vi "test_vision.vi"() -> ()   [LabVIEW 2011]
uses:
  Vision Instrumentation Control.ctl
  <vilib>/vision/NI_Vision_Development_Module.lvlib
panel:
  out "Exe Times":u32[](array[numeric])
  out "Total Execution Time":u32
  out "Avg Execution Time":dbl
  in  "Range":cluster{"Lower value":sgl, "Upper value":sgl}={"Lower value"=218.04347, "Upper value"=255.0} {"Lower value" scale=0.0..255.0; "Upper value" scale=0.0..255.0}
  in  "Score Limits":T1={"Rect Coverage"=76.0, "Aspect Ratio"=0.0, "X Edge Strength"=40.0, "Y Edge Strength"=50.0}
  in  "Area Size Limit":i32=444
  in  "Particle Count Limit":i32=8
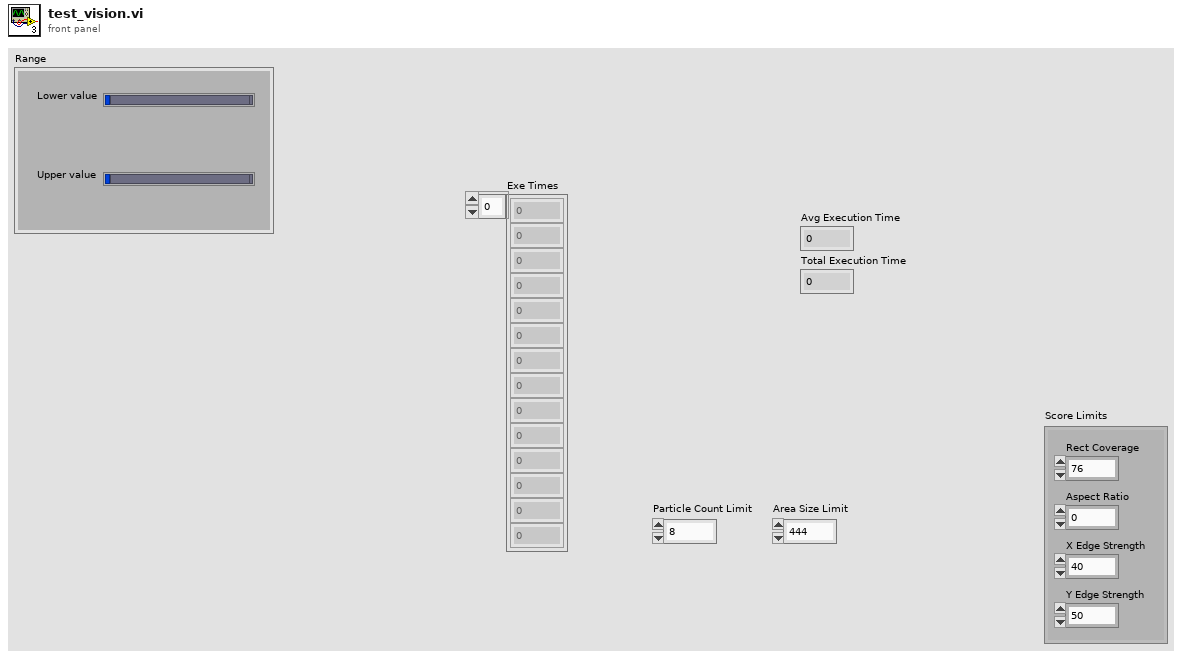
[diagram p1: front panel]
types:
  T1 = cluster{"Rect Coverage":dbl, "Aspect Ratio":dbl, "X Edge Strength":dbl, "Y Edge Strength":dbl}
  T2 = typedef "Image Type" = u32
  T3 = typedef "IMAQ Image.ctl" = refnum<image>
  T4 = typedef "Vision Instrumentation Control.ctl" = cluster{"Draw Boxes":bool, "Draw Scores":bool, "Draw Lines":bool, "Draw Line Angles":bool, "Draw Targets":bool, "Draw Compound Crosshair":bool, "Draw Center Line":bool}
  T5 = enum32{"AutoM", "Close", "Dilate", "Erode", "Gradient", "Gradient in", "Gradient out", "HitMiss", "Open", "PClose", "POpen", "Thick", "Thin"}
  T6 = enum32{"AutoM", "Close", "Dilate", "Erode", "Gradient", "Gradient out", "Gradient in", "Hit miss", "Open", "PClose", "POpen", "Thick", "Thin"}
  T7 = cluster{cluster{"Left":dbl, "Top":dbl, "Right":dbl, "Bottom":dbl}, cluster{"Score":dbl, "Score":dbl, "X Score":dbl, "Y Score":dbl}, "Clipped Edge":cluster{"Left":bool, "Top":bool, "Right":bool, "Bottom":bool}}[]
  T8 = typedef "Camera State.ctl" = enum16{"No Targets", "Low Confidence", "Medium Confidence", "High Confidence", "Camera Error"}
  T9 = cluster{"X Position":dbl, "Distance":dbl, "Camera State":T8}
  T10 = typedef "Diamond Target Output.ctl" = cluster{"Position":cluster{"X":dbl, "Y":dbl, "Distance":dbl}, "Est. Position":T11, "Target Confidence":T12}
  T11 = typedef "Rectangle Position.ctl" = enum16{"Unknown", "Top", "Right", "Left", "Bottom"}
  T12 = typedef "Target Confidence.ctl" = enum16{"Good", "Good-Clipped Y", "Marginal-Clipped X"}
  T13 = typedef "Line.ctl" = cluster{"First Point":cluster{"X":dbl, "Y":dbl, "Index":dbl}, "Second Point":cluster{"X":dbl, "Y":dbl, "Index":dbl}, "theta":dbl, "Direction":T14, "Line Confidence":T15}
  T14 = typedef "Direction.ctl" = enum16{"Rt", "Rt-Up", "Up", "Lt-Up", "Lt", "Lt-Dn", "Dn", "Rt-Dn", "Unknown"}
  T15 = typedef "Line Confidence.ctl" = enum16{"Good", "Bad"}
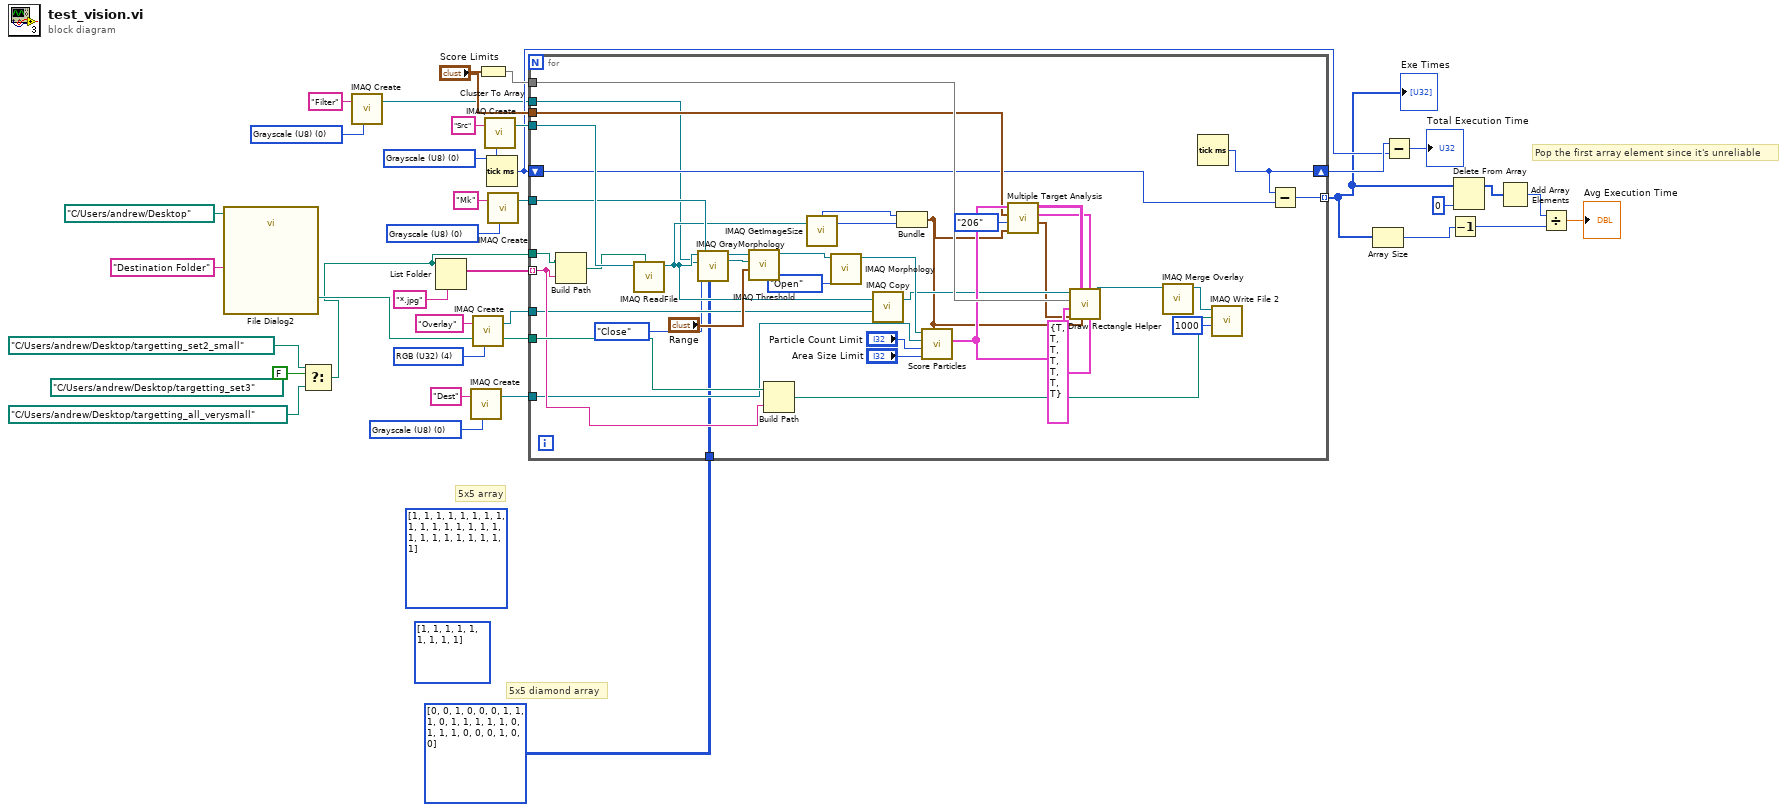
[diagram p0: block diagram]
diagram:
  (unwired) i32[][] [[1, 1, 1], [1, 1, 1], [1, 1, 1]] ("Structuring Element")
  (unwired) i32[][] [[1, 1, 1, 1, 1], [1, 1, 1, 1, 1], [1, 1, 1, 1, 1], [1, 1, 1, 1, 1], [1, 1, 1, 1, 1]] ("Structuring Element")
  w4 = T2 0 items=["Grayscale (U8)", "Grayscale (I16)", "Grayscale (SGL)", "Complex (CSG)", "RGB (U32)", "HSL (U32)", "RGB (U64)", "Grayscale (U16)"] ("Image Type")
  w17 = T2 4 items=["Grayscale (U8)", "Grayscale (I16)", "Grayscale (SGL)", "Complex (CSG)", "RGB (U32)", "HSL (U32)", "RGB (U64)", "Grayscale (U16)"] ("Image Type")
  (unwired) path "C:/Users/andrew/Desktop/targetting_set3" ("path")
  w23 = T2 0 items=["Grayscale (U8)", "Grayscale (I16)", "Grayscale (SGL)", "Complex (CSG)", "RGB (U32)", "HSL (U32)", "RGB (U64)", "Grayscale (U16)"] ("Image Type")
  w31 = T2 0 items=["Grayscale (U8)", "Grayscale (I16)", "Grayscale (SGL)", "Complex (CSG)", "RGB (U32)", "HSL (U32)", "RGB (U64)", "Grayscale (U16)"] ("Image Type")
  w33 = T2 0 items=["Grayscale (U8)", "Grayscale (I16)", "Grayscale (SGL)", "Complex (CSG)", "RGB (U32)", "HSL (U32)", "RGB (U64)", "Grayscale (U16)"] ("Image Type")
  # "5x5 diamond array"
  # "5x5 array"
  # "Pop the first array element since it's unreliable"
  n1 = call "File Dialog2"("start path"=path "C:/Users/andrew/Desktop", "prompt"="Destination Folder") -> ("selected path"=w27:path)  [unwired: 10 in, 3 out]
  n2 = Select(t=path "C:/Users/andrew/Desktop/targetting_set2_small" ("path"), s=FALSE, f=path "C:/Users/andrew/Desktop/targetting_all_verysmall" ("path")) -> (s? t:f=w20:path)
  n3 = call "IMAQ Create"("Image Name"="Filter", "Image Type"=w4) -> ("New Image"=w3:T3)  [unwired: 3 in, 1 out]
  n4 = List Folder(path=w20, pattern="*.jpg") -> (filenames=w35:string[])  [unwired: 2 in, 3 out]
  n5 = call "IMAQ Create"("Image Name"="Dest", "Image Type"=w23) -> ("New Image"=w24:T3)  [unwired: 3 in, 1 out]
  n6 = call "IMAQ Create"("Image Name"="Overlay", "Image Type"=w17) -> ("New Image"=w16:T3)  [unwired: 3 in, 1 out]
  n7 = Cluster To Array(cluster="Score Limits") -> (array=w28:dbl[])
  n8 = call "IMAQ Create"("Image Name"="Src", "Image Type"=w33) -> ("New Image"=w30:T3)  [unwired: 3 in, 1 out]
  n9 = Tick Count (ms)() -> (millisecond timer value=w12:u32)
  n10 = call "IMAQ Create"("Image Name"="Mk", "Image Type"=w31) -> ("New Image"=w29:T3)  [unwired: 3 in, 1 out]
  n11 = for {
    tunnel: w35 -> [w60] mode=indexing
    tunnel: w30 -> [w75]
    tunnel: w20 -> [w73]
    tunnel: w29 -> [w72]
    tunnel: w28 -> [w62]
    tunnel: w27 -> [w61]
    tunnel: w24 -> [w59]
    tunnel: "Score Limits" -> [w57]
    tunnel: w16 -> [w50]
    shift-right: [w46] -> w13
    shift-left: w12 -> [w45]
    tunnel: [w44] -> w10 mode=indexing
    tunnel: w3 -> [w41]
    tunnel: i32[][] [[0, 0, 1, 0, 0], [0, 1, 1, 1, 0], [1, 1, 1, 1, 1], [0, 1, 1, 1, 0], [0, 0, 1, 0, 0]] ("Structuring Element") -> [w39]
    n12 = Build Path(base path=w73, name or relative path=w60) -> (appended path=w74:path)
    n13 = call "IMAQ ReadFile"("File Path"=w74, "Image"=w75) -> ("Image Out"=w42:T3)  [unwired: 5 in, 4 out]
    n14 = call "IMAQ GrayMorphology"("Structuring Element"=w39, "Operation"=T5."Close", "Image Dst"=w41, "Image Src"=w42) -> ("Image Dst Out"=w43:T3)  [unwired: 6 in, 1 out]
    n15 = call "IMAQ Threshold"("Range"="Range", "Image Dst"=w72, "Image Src"=w43) -> ("Image Dst Out"=w71:T3)  [unwired: 7 in, 1 out]
    n16 = Build Path(base path=w61, name or relative path=w60) -> (appended path=w66:path)
    n17 = call "IMAQ GetImageSize"("Image"=w42) -> ("Y Resolution"=w51:i32, "X Resolution"=w52:i32)  [unwired: 3 in, 1 out]
    n18 = call "IMAQ Morphology"("Operation"=T6."Open", "Image Src"=w71) -> ("Image Dst Out"=w67:T3)  [unwired: 8 in, 1 out]
    n19 = call "IMAQ Copy"("Image Dst"=w50, "Image Src"=w42) -> ("Image Dst Out"=w49:T3)  [unwired: 4 in, 1 out]
    n20 = Bundle("X Resolution"=w52, "Y Resolution"=w51) -> (w47:cluster{"X Resolution":i32, "Y Resolution":i32})  [unwired: 1 in]
    n21 = call "Score Particles.vi"("Image Size"=w47, "Area Size Limit"="Area Size Limit", "Particle Count Limit"="Particle Count Limit", "Image Dst"=w59, "Image Refnum in"=w67) -> ("Targets"=w58:T7)  [unwired: 5 in, 1 out]
    n22 = call "Multiple Target Analysis.vi"("Image Size"=w47, "Camera Type"=enum16{"206", "1011"}."206", "Score Limits"=w57, "Targets"=w58) -> ("Targetting Output"=w48:T9, "Diamond Targets"=w54:T10[], "Lines"=w55:T13[][])  [unwired: 5 in]
    n23 = call "Draw Rectangle Helper.vi"("Vision Instrumentation"=T4 {"Draw Boxes"=TRUE, "Draw Scores"=TRUE, "Draw Lines"=TRUE, "Draw Line Angles"=TRUE, "Draw Targets"=TRUE, "Draw Compound Crosshair"=TRUE, "Draw Center Line"=TRUE}, "Diamond Targets"=w54, "Image Size"=w47, "Lines"=w55, "Targetting Output"=w48, "Targets"=w58, "Score Limits"=w62, "Refnum in"=w49) -> ("Refnum out"=w64:T3)  [unwired: 3 in]
    n24 = call "IMAQ Merge Overlay"("Image Src"=w64) -> ("Image Dst Out"=w63:T3)  [unwired: 9 in, 1 out]
    n25 = Tick Count (ms)() -> (millisecond timer value=w46:u32)
    n26 = call-poly "IMAQ Write File 2"("Image Quality"=u32 1000, "File Path"=w66, "Image"=w63) -> ()  [unwired: 7 in, 2 out]
    n27 = Subtract(x=w46, y=w45) -> (x-y=w44:u32)
  }
  "Exe Times" <- w10
  n28 = Array Size(array=w10) -> (size(s)=w7:i32)
  n29 = Subtract(x=w13, y=w12) -> (x-y=→"Total Execution Time":u32)
  n30 = Decrement(x=w7) -> (x-1=w6:i32)
  n31 = Delete From Array(array=w10, index=0) -> (array with subset deleted=w9:u32[])  [unwired: 1 in, 1 out]
  n32 = Add Array Elements(numeric array=w9) -> (sum=w15:u32)
  n33 = Divide(x=w15, y=w6) -> (x/y=→"Avg Execution Time":dbl)
